vi "MEC751 Final VI cleaned up.vi"() -> ()   [LabVIEW 2013]
uses:
  <vilib>/express/express analysis/Spectral/Block/exnSpectralBlock spectral measurements RMS poly.vi
  <vilib>/express/express analysis/Spectral/Block/exnSpectralBlock spectral measurements RMS DDT.vi
  <vilib>/express/express analysis/Spectral/XNode/ExpressSpectralMeasurementsBlockNode.xnode
panel:
  out "Overload":bool
  out "0/0":bool
  out "Error":dbl
  out "Deadzone":bool
  out "POT Gram reading":dbl
  out "Reverse Voltage":dbl
  out "Done":bool
  in  "POT Gram Start Deadzone":dbl
  out "Pot Vout Value":dbl
  in  "Max POT Voltage":dbl
  out "DC Out":dynamicdata(graph)
  out "Voltage out to Motor":dbl
  out "Modified Error":dbl
  in  "Differential Gain":dbl
  in  "Proportional Gain":dbl
  out "Gram Input":dbl
  out "POT Vout":dynamicdata(graph)
  out "Mass":dbl(graph)
  out "sens":dbl format="%_8g"
  in  "cali. mass":dbl format="%_8g"
  in  "Slope":bool
  out "V2":dbl format="%_8g"
  out "V1":dbl format="%_8g"
  out "Mass (kg)":dbl format="%_8g"
  in  "1st mass for calibration (kg) (0 preferred) 2":dbl
  in  "Tare":bool
  in  "number of samples":i32=100
  in  "rate":dbl=1000.0
  out "Avg. V (V)":dbl format="%_8g"
  out "fft":dynamicdata(graph)
  out "Voltage":dynamicdata(graph)
  in  "stop (F)":bool
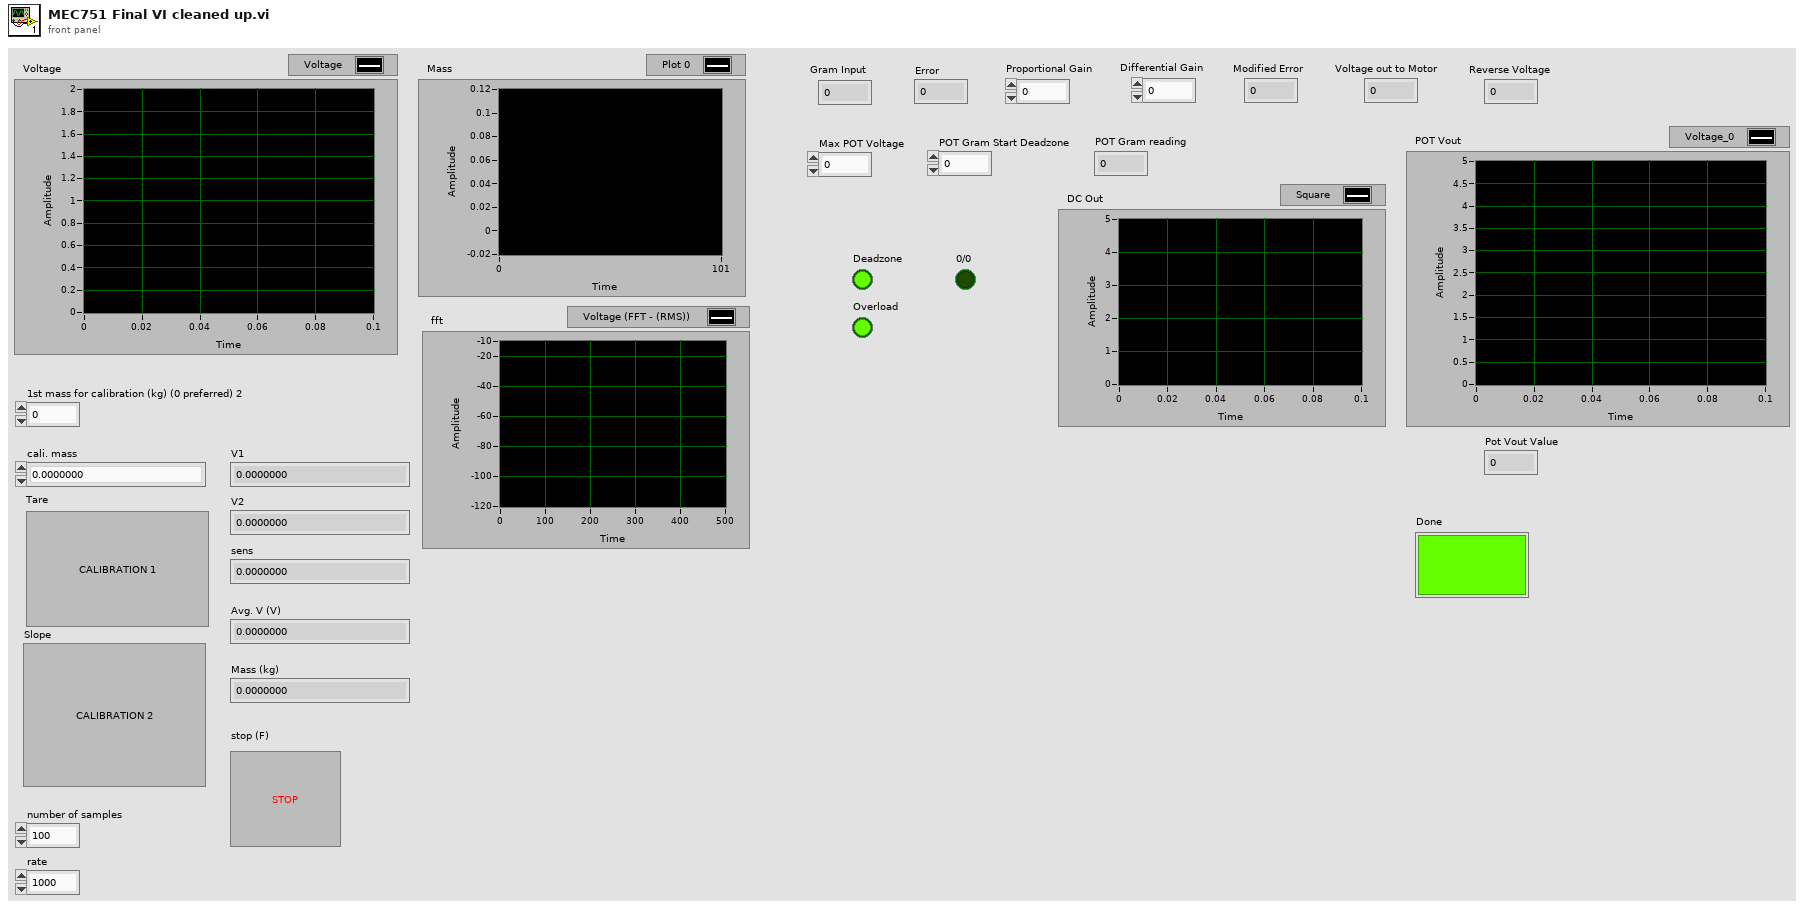
[diagram p1: front panel]
types:
  T1 = cluster{"averaging mode":u16, "weighting mode":u16, "number of averages":u32}
  T2 = cluster{"dB On (F)":bool, "unwrap phase (F)":bool, "convert to degree (F)":bool}
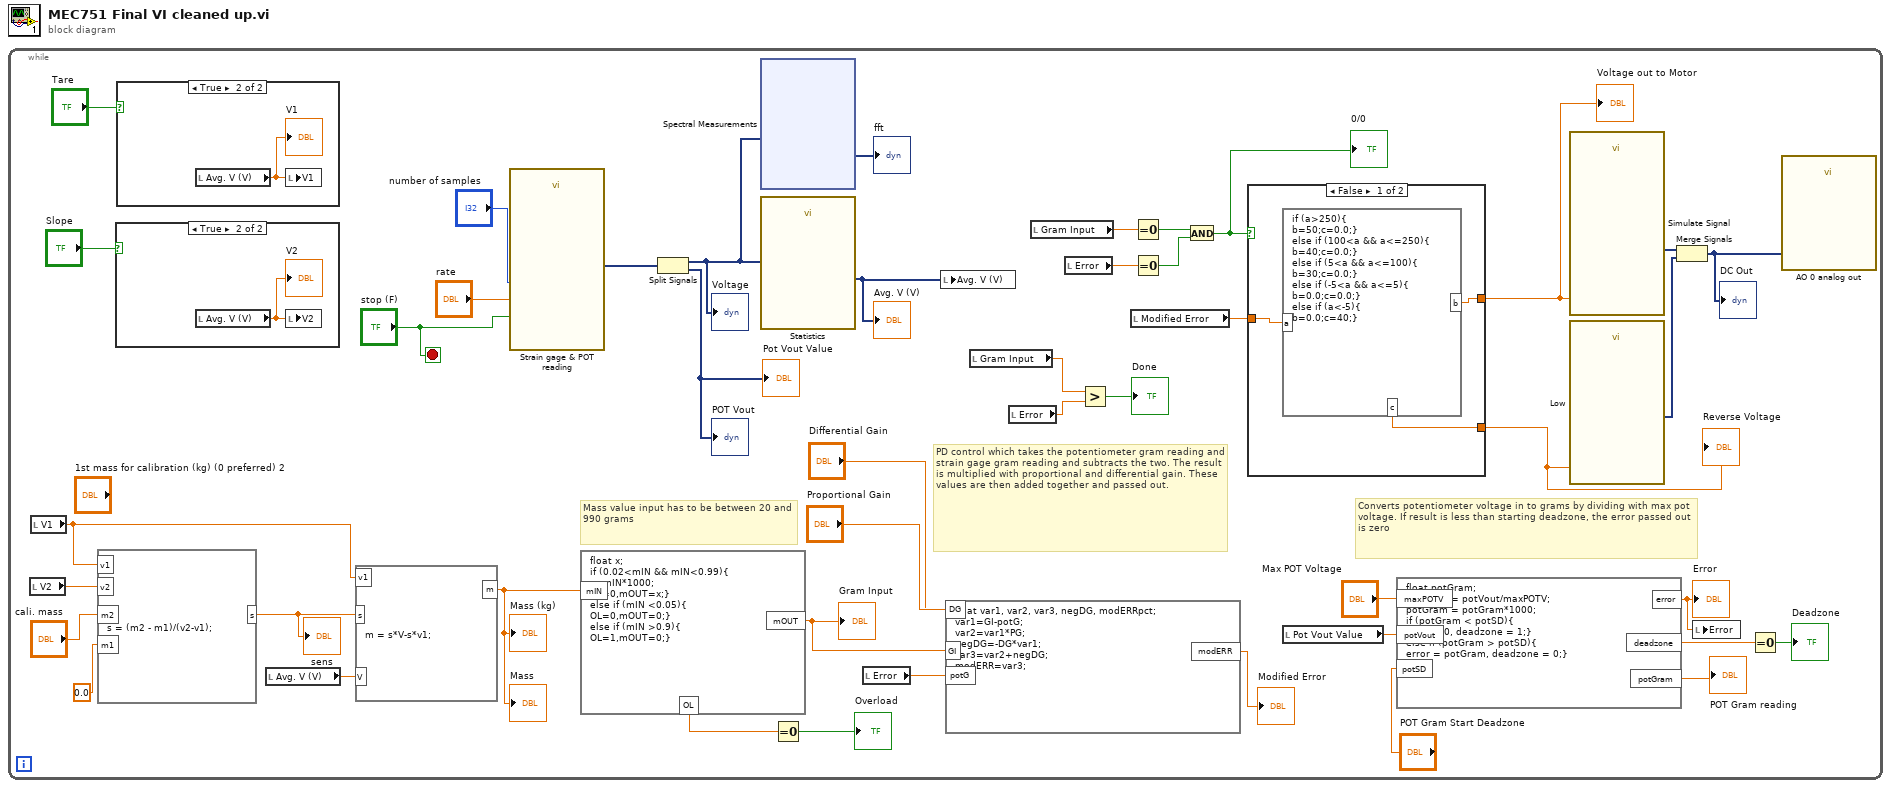
[diagram p0: block diagram]
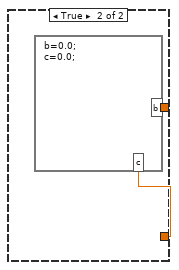
[diagram p2: hidden frame]
diagram:
  n1 = while {
    stop <- "stop (F)" stop-if-true
    # "PD control which takes the potentiometer gram reading and strain gage gram reading and subtracts the two. The result is multiplied with proportional and differential gain. These values are then added together and passed out."
    # "Converts potentiometer voltage in to grams by dividing with max pot voltage. If result is less than starting deadzone, the error passed out is zero"
    # "Mass value input has to be between 20 and 990 grams"
    n2 = local read "V2"() -> (w38:dbl)
    n3 = local read "V1"() -> (w34:dbl)
    n4 = formula code="s = (m2 - m1)/(v2-v1);"("v1"=w34, "m2"="cali. mass", "m1"=0.0 ("input variable"), "v2"=w38) -> ("s"=w35:dbl)
    "sens" <- w35
    n5 = case shown="True" "Slope" {
      frame False {
      }
      frame True {
        n6 = local read "Avg. V (V)"() -> (w51:dbl)
        "V2" <- w51
        n7 = local write "V2"(w51) -> ()
      }
    }
    n8 = case shown="True" "Tare" {
      frame False {
      }
      frame True {
        n9 = local read "Avg. V (V)"() -> (w52:dbl)
        "V1" <- w52
        n10 = local write "V1"(w52) -> ()
      }
    }
    n11 = local read "Avg. V (V)"() -> (w37:dbl)
    n12 = formula code="m = s*V-s*v1;"("s"=w35, "V"=w37, "v1"=w34) -> ("m"=w21:dbl)
    "Mass (kg)" <- w21
    "Mass" <- w21
    n13 = call "Strain gage & POT reading"("rate"="rate", "number of samples"="number of samples", "stop (T)"="stop (F)") -> ("data"=w33:dynamicdata)  [unwired: 14 in, 2 out]
    n14 = formula code="float x;\nif (0.02<mIN && mIN<0.99){\nx=mIN*1000;\nOL=0,mOUT=x;}\nelse if (mIN <0.05){\nOL=0,mOUT=0;}\nelse if (mIN >0.9){\nOL=1,mOUT=0;}"("mIN"=w21) -> ("mOUT"=w2:dbl, "OL"=w20:dbl)
    "Gram Input" <- w2
    n15 = Split Signals(w33) -> (w32:dynamicdata, →"POT Vout" →"Pot Vout Value":dynamicdata)  [unwired: 2 in]
    "Voltage" <- w32
    n16 = xnode "Spectral Measurements"("Signals"=w32) -> ("FFT - (RMS)"=→"fft":dynamicdata)  [unwired: 2 in, 3 out]
    n17 = call "Statistics"("Signals"=w32) -> ("Arithmetic Mean"=w36:dynamicdata)  [unwired: 25 in, 1 out]
    "Avg. V (V)" <- w36
    n18 = Equal To 0?(x=w20) -> (x = 0?=→"Overload":bool)
    n19 = local read "Error"() -> (w16:dbl)
    n20 = local write "Avg. V (V)"(w36) -> ()
    n21 = formula code="float var1, var2, var3, negDG, modERRpct;\nvar1=GI-potG;\nvar2=var1*PG;\nnegDG=-DG*var1;\nvar3=var2+negDG;\nmodERR=var3;"("GI"=w2, "PG"="Proportional Gain", "DG"="Differential Gain", "potG"=w16) -> ("modERR"=→"Modified Error":dbl)
    n22 = local read "Gram Input"() -> (w3:dbl)
    n23 = local read "Error"() -> (w4:dbl)
    n24 = local read "Gram Input"() -> (w25:dbl)
    n25 = local read "Error"() -> (w24:dbl)
    n26 = Greater?(x=w3, y=w4) -> (0:→"Done":bool)
    n27 = local read "Modified Error"() -> (w28:dbl)
    n28 = Equal To 0?(x=w25) -> (x = 0?=w23:bool)
    n29 = Equal To 0?(x=w24) -> (x = 0?=w22:bool)
    n30 = And(x=w23, y=w22) -> (x .and. y?=w15:bool)
    "0/0" <- w15
    n31 = case shown="False" w15 {
      tunnel: w28 -> [w48 _]
      tunnel: [w47 w49] -> w6
      tunnel: [w46 w50] -> w1
      frame False {
        n32 = formula code="if (a>250){\nb=50;c=0.0;}\nelse if (100<a && a<=250){\nb=40;c=0.0;}\nelse if (5<a && a<=100){\nb=30;c=0.0;}\nelse if (-5<a && a<=5){\nb=0.0;c=0.0;}\nelse if (a<-5){\nb=0.0;c=40;}"("a"=w48) -> ("b"=w47:dbl, "c"=w46:dbl)
      }
      frame True {
        n33 = formula code="b=0.0;\nc=0.0;"() -> ("b"=w49:dbl, "c"=w50:dbl)
      }
    }
    "Voltage out to Motor" <- w6
    "Reverse Voltage" <- w1
    n34 = local read "Pot Vout Value"() -> (w9:dbl)
    n35 = formula code="float potGram;\npotGram = potVout/maxPOTV;\npotGram = potGram*1000;\nif (potGram < potSD){\nerror = 0, deadzone = 1;}\nelse if (potGram > potSD){\nerror = potGram, deadzone = 0;}"("maxPOTV"="Max POT Voltage", "potVout"=w9, "potSD"="POT Gram Start Deadzone") -> ("error"=w7:dbl, "deadzone"=w14:dbl, "potGram"=→"POT Gram reading":dbl)
    "Error" <- w7
    n36 = call "Simulate Signal"("Duty Cycle (%)"=w6) -> ("Square"=w31:dynamicdata)  [unwired: 13 in, 1 out]
    n37 = call "Low"("Duty Cycle (%)"=w1) -> ("Square"=w30:dynamicdata)  [unwired: 13 in, 1 out]
    n38 = Merge Signals(w31, w30) -> (w29:dynamicdata)
    "DC Out" <- w29
    n39 = local write "Error"(w7) -> ()
    n40 = Equal To 0?(x=w14) -> (x = 0?=→"Deadzone":bool)
    n41 = call "AO 0 analog out"("data"=w29) -> ()  [unwired: 17 in, 2 out]
  }
